vi "Is prime-v2.vi"(8 "error in (no error)":errorcluster, 10 "List of all prime numbers smaller than x":i32[](array[numeric])=[2, 3, 5, 7, 11], 11 "x":i32=13) -> (0 "error out":errorcluster, 3 "T = is prime":bool)   [LabVIEW 2021, in "Numeric Utilities.lvlib"]
uses:
  Numeric Utilities.lvlib
panel:
  # "Development\ncontrols/indicators useful for development and testing, but which are not outputs of the VI"
  # "Input\nInputs to the VI"
  # "Output\nOutputs of the VI"
  # "Description\n\nBlank VI with error handling case. \n\nSummarize the use of this VI in this space."
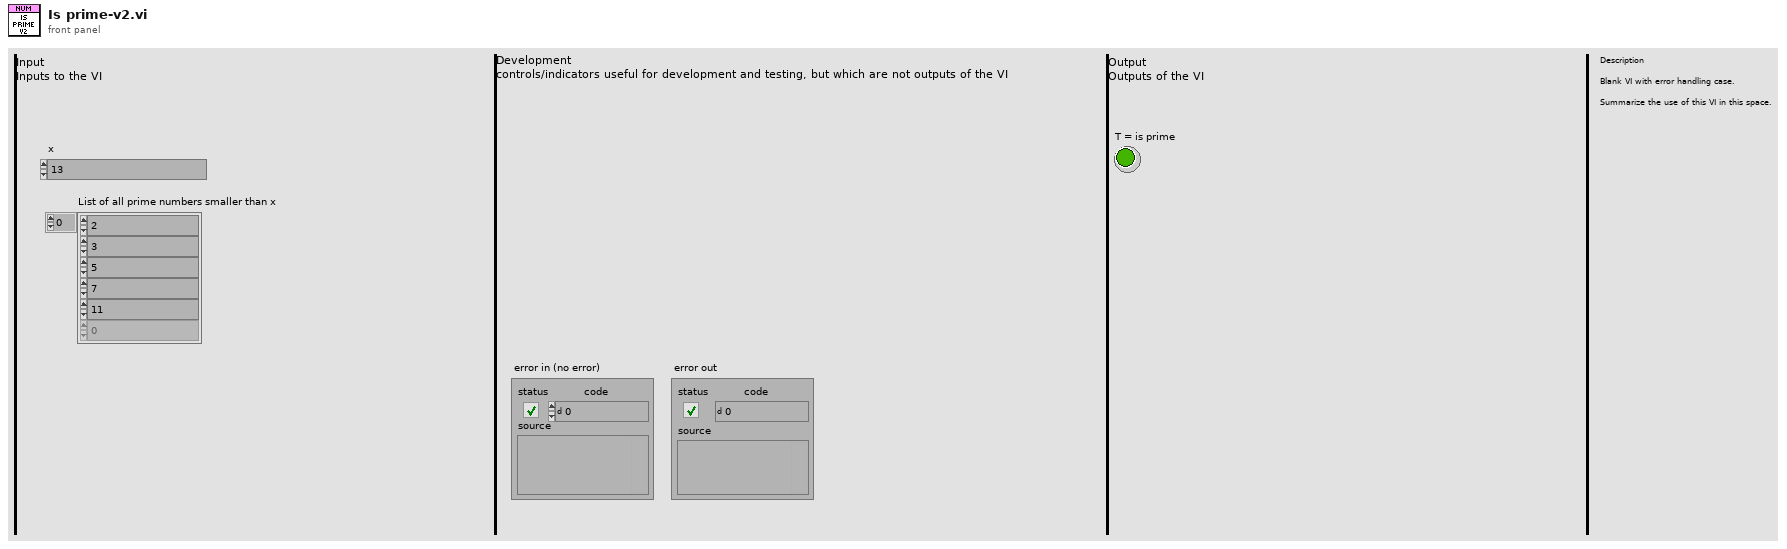
[diagram p1: front panel]
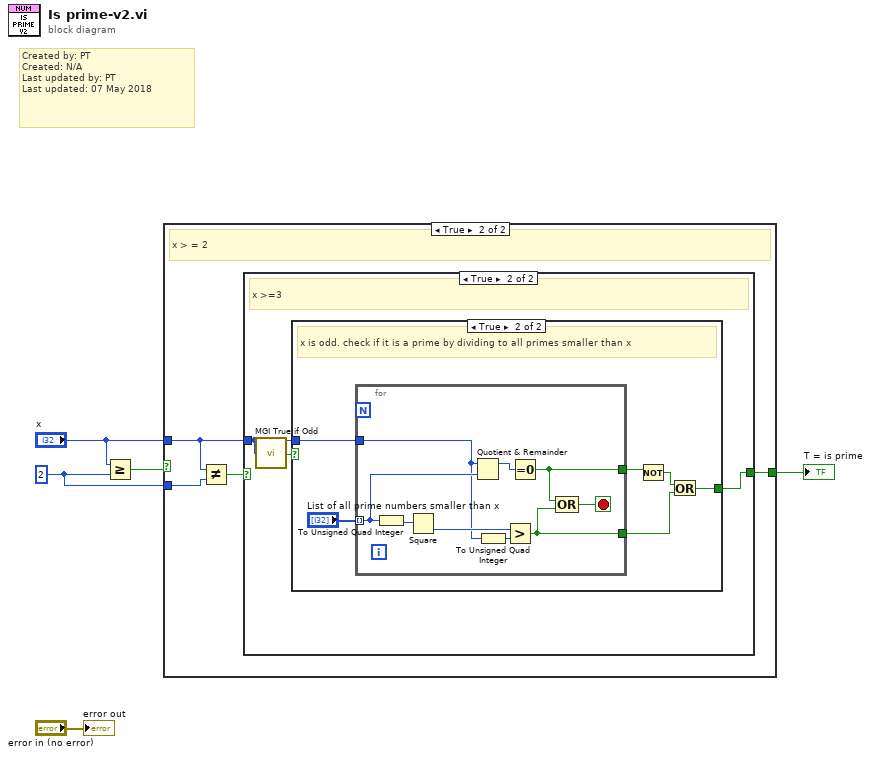
[diagram p0: block diagram]
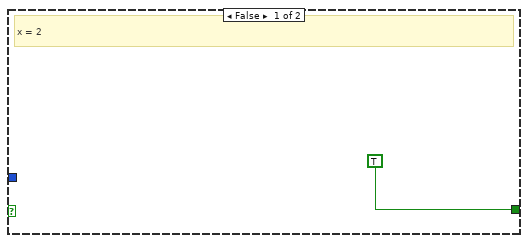
[diagram p3: hidden frame]
diagram:
  w1 = 2 ("y")
  # "Created by: PT\nCreated: N/A\nLast updated by: PT\nLast updated: 07 May 2018"
  n1 = Greater Or Equal?(x="x", y=w1) -> (x >= y?=w2:bool)
  n2 = case shown="True" w2 {
    tunnel: "x" -> [_ w8]
    tunnel: [_ w9] -> w4
    tunnel: w1 -> [_ w7]
    frame False {
      # "x is 0 or 1"
    }
    frame True {
      # "x > = 2"
      n3 = Not Equal?(x=w8, y=w7) -> (x != y?=w6:bool)
      n4 = case shown="True" w6 {
        tunnel: w8 -> [_ w12]
        tunnel: [TRUE w13] -> w9
        frame False {
          # "x = 2"
        }
        frame True {
          # "x >=3"
          n5 = call <userlib>:"MGI True if Odd.vi"("Integer"=w12) -> ("Odd?"=w11:bool)
          n6 = case shown="True" w11 {
            tunnel: w12 -> [_ w19]
            tunnel: [_ w14] -> w13
            frame False {
              # "x is even and >=3. x cannot be a prime"
            }
            frame True {
              # "x is odd. check if it is a prime by dividing to all primes smaller than x"
              n7 = for {
                tunnel: w19 -> [w24]
                tunnel: [w27] -> w18
                tunnel: "List of all prime numbers smaller than x" -> [w26] mode=indexing
                tunnel: [w20] -> w15
                stop <- w23 stop-if-true
                n8 = To Unsigned Quad Integer(1:w26) -> (0:w22:u64)
                n9 = Square(x=w22) -> (x^2=w25:u64)
                n10 = Quotient & Remainder(x=w24, y=w26) -> (x-y*floor(x/y)=w28:i32)  [unwired: 1 out]
                n11 = To Unsigned Quad Integer(1:w24) -> (0:w21:u64)
                n12 = Greater?(x=w25, y=w21) -> (0:w20:bool)
                n13 = Equal To 0?(x=w28) -> (x = 0?=w27:bool)
                n14 = Compound Arithmetic op=OR(w27, w20) -> (w23:bool)
              }
              n15 = Not(x=w18) -> (.not. x?=w16:bool)
              n16 = Or(x=w16, y=w15) -> (x .or. y?=w14:bool)
            }
          }
        }
      }
    }
  }
  "T = is prime" <- w4
  "error out" <- "error in (no error)"
